vi "Rad to Deg(dbl)L.vi"(1 "radian":dbl) -> (0 "degree":dbl)   [LabVIEW 2012, in "几何工具.lvlib"]
doc: "功能：\n\n弧度转换为角度。\n\n输入：弧度。\n\n输出：角度，单位为度。\n\ncsxcs_366创建。"
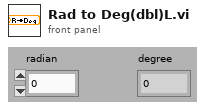
[diagram p1: front panel]
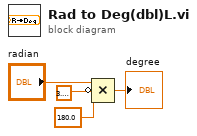
[diagram p0: block diagram]
diagram:
  n1 = Compound Arithmetic op=MULTIPLY("radian", invert 3.141592653589793, 180.0 ("值")) -> (→"degree":dbl)
